vi "Main.vi"() -> ()   [LabVIEW 2014]
doc: "The boiler controller allows a user to start and shut down a boiler.\n\nUse the Reset, Start, and Light Pilot controls to sequentially start the boiler. \nUse the Fuel Control Valve to change the flow of fuel into the boiler. \nUse the Stop Boiler button to shut down the boiler. \nTo shut down the system or in the event of an emergency, use the Emergency Stop button to close the application completely."
uses:
  controls/MHL Data.ctl
  controls/MHL UI Data.ctl
  controls/MHL Status.ctl
  controls/MHL References.ctl
  controls/MHL Configuration.ctl
  support/Boiler System Globals.vi
  <vilib>/Utility/error.llb/Error Cluster From Error Code.vi
  <vilib>/ErrorRing/Error Ring.xnode
  support/Message Queue/Message Queue.lvlib
  support/User Event - Stop/User Event - Stop.lvlib
  Boiler/Boiler.lvlib
panel:
  in  "Fuel Control Valve":u32(slide) min=10 max=75 scale=10.0..75.0
  in  "Stop Boiler":bool
  in  "Light Pilot":bool
  out "Forced Draft Fan":bool
  out "Pilot":bool
  out "Pilot Gas Valve":bool
  out "Primary Fan":bool
  out "Status":string
  in  "Start":bool
  in  "Reset":bool
  in  "Emergency Stop":bool
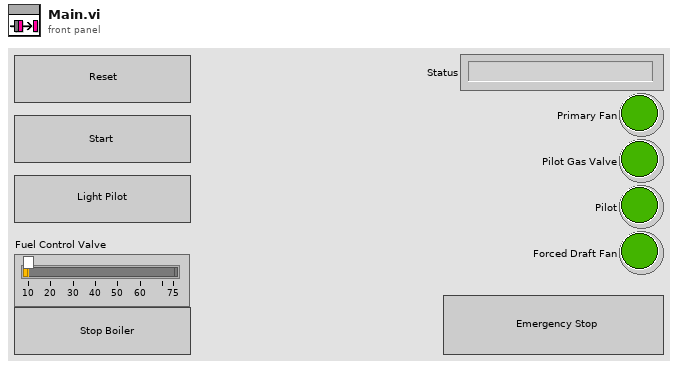
[diagram p1: front panel]
types:
  T1 = typedef "MHL Data.ctl" = cluster{"MHL User Interface Data":T2, "MHL References":T4, "MHL Configuration":T5}
  T2 = typedef "MHL UI Data.ctl" = cluster{"Status":string, "Fuel Control Valve":u32, "Primary Fan":bool, "Pilot Gas Valve":bool, "Pilot":bool, "Forced Draft Fan":bool, "MHL Status":T3}
  T3 = typedef "MHL Status.ctl" = enum16{"Lockout", "Ready", "Pre-Purge", "Pre-Purge Complete", "Pilot On", "Boiler Running", "Shutdown", "Purge"}
  T4 = typedef "MHL References.ctl" = cluster{"Reset Ref":refnum<vi>, "Start Ref":refnum<vi>, "Light Pilot Ref":refnum<vi>, "Stop Boiler Ref":refnum<vi>, "Fuel Control Valve Ref":refnum<vi>}
  T5 = typedef "MHL Configuration.ctl" = cluster{"Fuel Control Valve Maximum":dbl, "Fuel Control Valve Minimum":dbl}
  T6 = typedef "Notifiers.ctl" = cluster{"Handshake":refnum<notifier>, "Flame Level":refnum<notifier>, "Controller Exit":refnum<notifier>, "Boiler Exit":refnum<notifier>}
  T7 = typedef "Message Queue.lvlib/All Message Queues.ctl" = cluster{"MHL":refnum<queue>, "Boiler Controller":refnum<queue>, "Boiler":refnum<queue>}
  T8 = enum16{"open", "replace", "create", "open or create", "replace or create", "replace or create with confirmation"}
  T9 = enum32{"invalid app kind", "Development System", "Run Time System", "Student Edition", "Embedded LabVIEW", "Evaluation", "Custom"}
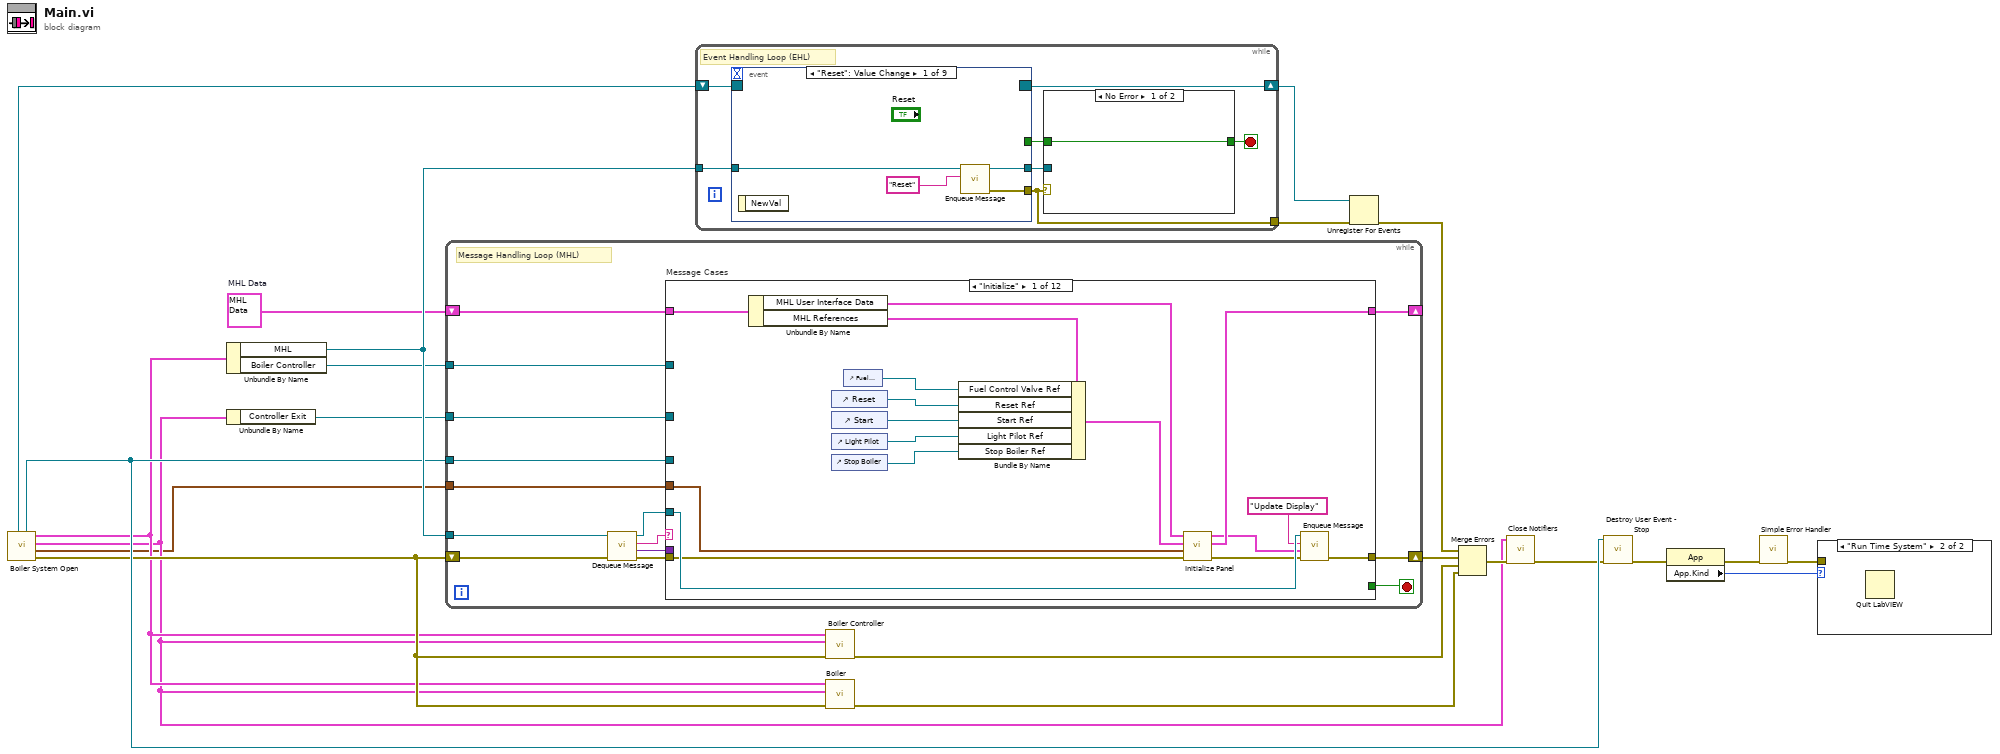
[diagram p0: block diagram]
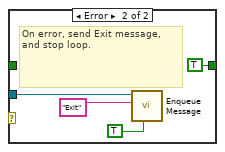
[diagram p3: hidden frame]
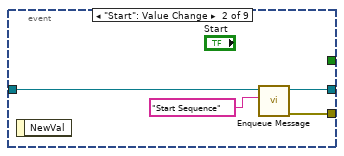
[diagram p4: hidden frame]
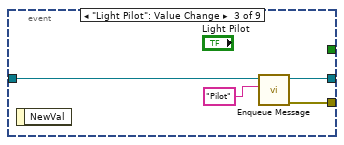
[diagram p5: hidden frame]
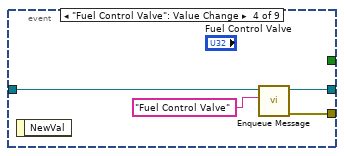
[diagram p6: hidden frame]
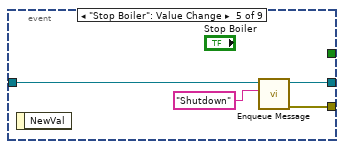
[diagram p7: hidden frame]
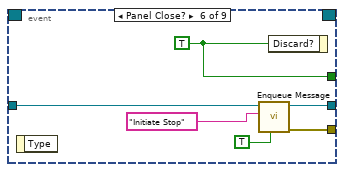
[diagram p8: hidden frame]
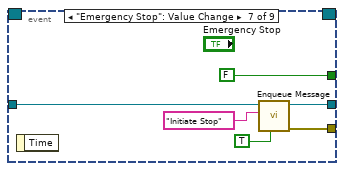
[diagram p9: hidden frame]
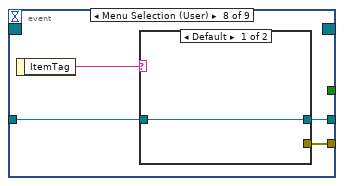
[diagram p10: hidden frame]
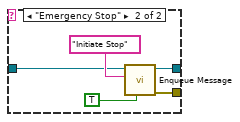
[diagram p11: hidden frame]
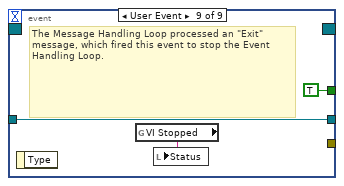
[diagram p12: hidden frame]
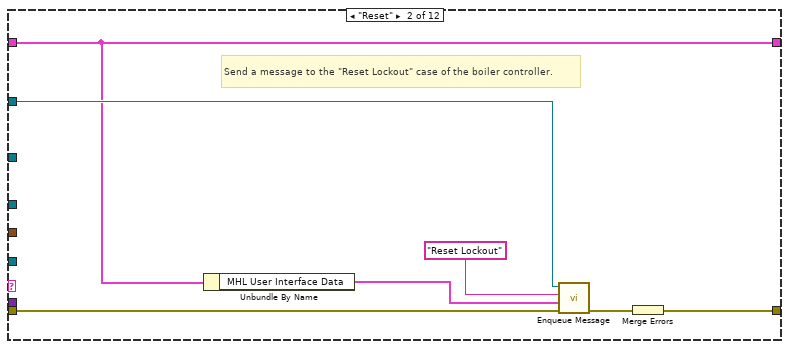
[diagram p13: hidden frame]
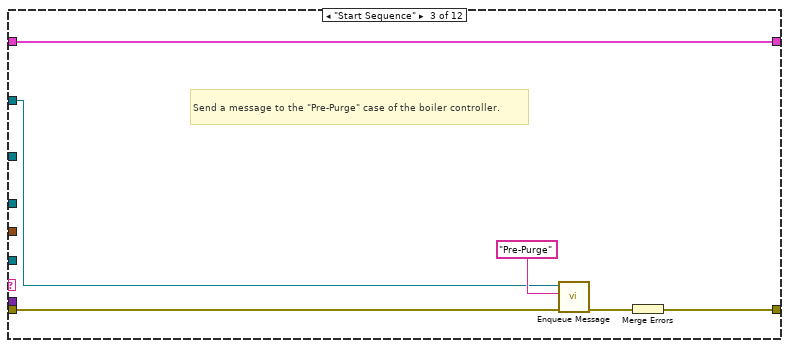
[diagram p14: hidden frame]
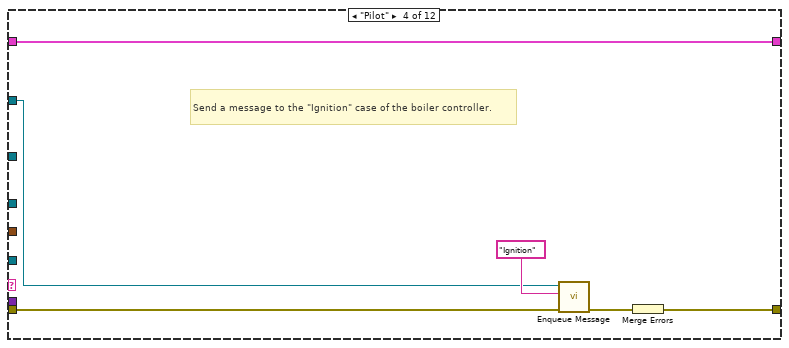
[diagram p15: hidden frame]
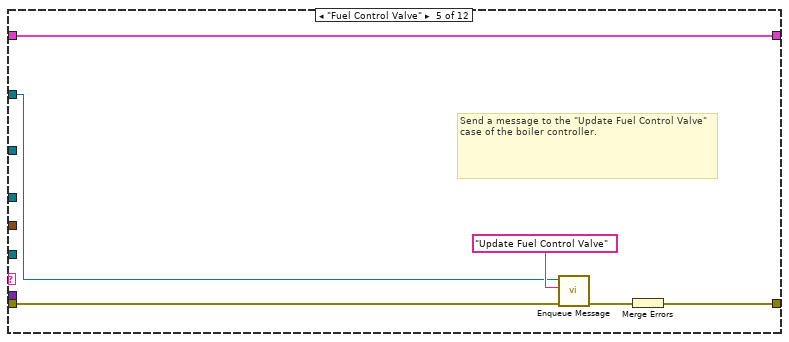
[diagram p16: hidden frame]
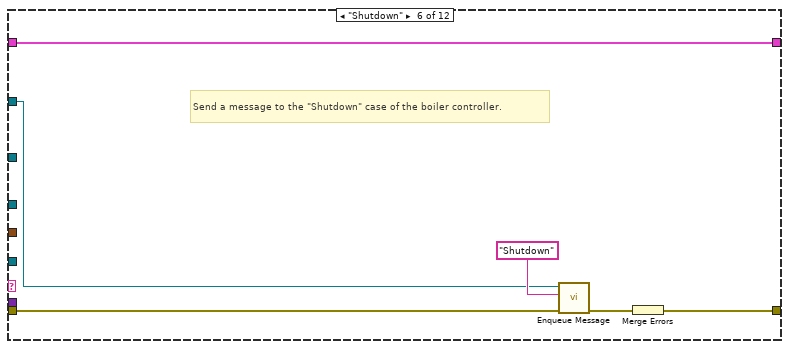
[diagram p17: hidden frame]
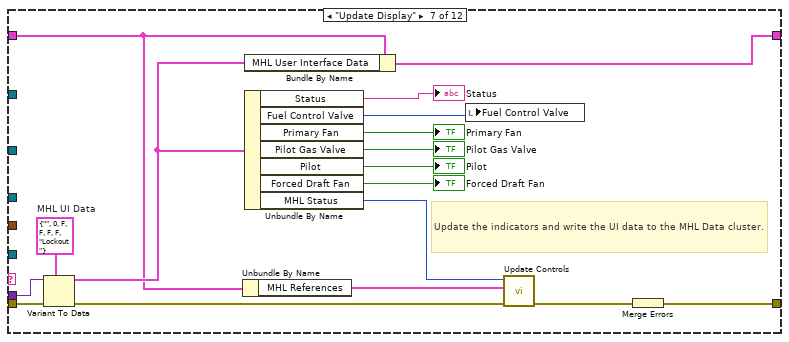
[diagram p18: hidden frame]
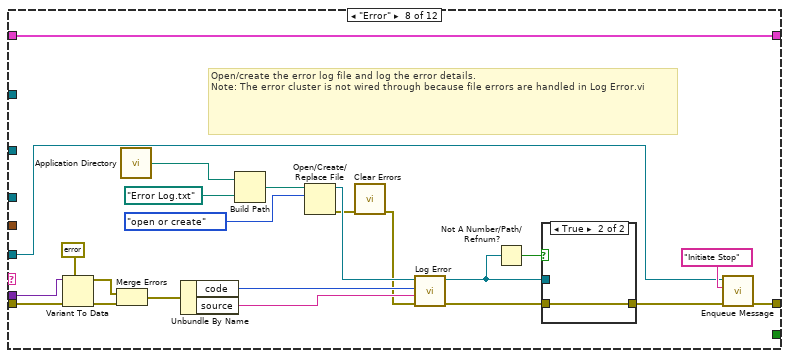
[diagram p19: hidden frame]
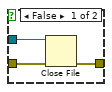
[diagram p20: hidden frame]
diagram:
  w16 = T1 {"MHL User Interface Data"={"Status"="", "Fuel Control Valve"=0, "Primary Fan"=FALSE, "Pilot Gas Valve"=FALSE, "Pilot"=FALSE, "Forced Draft Fan"=FALSE, "MHL Status"=enum."Lockout"}, "MHL References"={"Reset Ref"=refnum, "Start Ref"=refnum, "Light Pilot Ref"=refnum, "Stop Boiler Ref"=refnum, "Fuel Control Valve Ref"=refnum}, "MHL Configuration"={"Fuel Control Valve Maximum"=0.0, "Fuel Control Valve Minimum"=0.0}}  # MHL Data
  n1 = call "Boiler System Open.vi"() -> ("error out"=w7:errorcluster, "MHL Configuration"=w1:T5, "Notifiers"=w2:T6, "Message Queues"=w6:T7, "User Event - Stop"=w9:refnum<user-event>, "Stop Event Registration Refnum"=w10:refnum<event-registration>)  [unwired: 6 in]
  n2 = Unbundle By Name(w6) -> ("MHL"=w21:refnum<queue>, "Boiler Controller"=w14:refnum<queue>)
  n3 = Unbundle By Name(w2) -> ("Controller Exit"=w8:refnum<notifier>)
  n4 = while {
    tunnel: w21 -> [w26]
    shift-right: [w35] -> _
    shift-left: w16 -> [w36]
    tunnel: w9 -> [w32]
    shift-right: [w33] -> w22
    shift-left: w7 -> [w31]
    tunnel: w14 -> [w25]
    tunnel: w8 -> [w24]
    tunnel: w1 -> [w23]
    stop <- w34 stop-if-true
    # "Message Handling Loop (MHL)"
    n5 = call "Dequeue Message.vi"("error in (no error)"=w31, "Message Queue"=w26) -> ("error out"=w30:errorcluster, "Message Data"=w28:variant, "Message"=w29:string, "dup Message Queue"=w27:refnum<queue>)  [unwired: 6 in]
    n6 = case "Message Cases" shown="\"Initialize\"" w29 {
      selector: w29 -> [_ _ _ _ _ _ _ _ _ _ _ w162]
      tunnel: w27 -> [w46 _ _ _ _ _ _ w110 w131 w138 w160 _]
      tunnel: w30 -> [w40 w59 w64 w70 w73 w82 w100 w108 w136 w140 w153 _]
      tunnel: [w47 w60 w65 w71 w78 w83 w101 w106 w133 w139 w156 w161] -> w33
      tunnel: w36 -> [w48 w55 w66 w72 w74 w84 w86 w124 w135 w144 w159 w163]
      tunnel: [w38 w55 w66 w72 w74 w84 w90 w124 w135 w144 w159 w163] -> w35
      tunnel: [_ _ _ _ _ _ _ _ _ _ TRUE _] -> w34
      tunnel: w28 -> [_ _ _ _ _ _ w99 w107 _ _ _ _]
      tunnel: w32 -> [_ _ _ _ _ _ _ _ _ _ w155 _]
      tunnel: w25 -> [_ w56 w61 w67 w75 w79 _ _ w132 _ _ _]
      tunnel: w24 -> [_ _ _ _ _ _ _ _ _ w137 _ _]
      tunnel: w23 -> [w44 _ _ _ _ _ _ _ _ _ _ _]
      frame "Initialize" {
        n7 = Unbundle By Name(w48) -> ("MHL User Interface Data"=w41:T2, "MHL References"=w42:T4)
        n8 = control-ref of="Reset"() -> (w50:refnum<vi>)
        n9 = control-ref of="Start"() -> (w51:refnum<vi>)
        n10 = control-ref of="Light Pilot"() -> (w52:refnum<vi>)
        n11 = control-ref of="Stop Boiler"() -> (w53:refnum<vi>)
        n12 = control-ref of="Fuel Control Valve"() -> (w49:refnum<vi>)
        n13 = Bundle By Name(cluster=w42, "Fuel Control Valve Ref"=w49, "Reset Ref"=w50, "Start Ref"=w51, "Light Pilot Ref"=w52, "Stop Boiler Ref"=w53) -> (w43:T4)
        n14 = call "Initialize Panel.vi"("error in"=w40, "MHL Configuration"=w44, "MHL References"=w43, "MHL UI Data in"=w41) -> ("error out"=w39:errorcluster, "MHL Data out"=w38:T1, "MHL UI Data out"=w37:T2)  [unwired: 5 in]
        n15 = call "Enqueue Message.vi"("error in (no error)"=w39, "Message Data"=w37, "Message"="Update Display", "Message Queue"=w46) -> ("error out"=w47:errorcluster)  [unwired: 6 in, 1 out]
      }
      frame "Reset" {
        # "Send a message to the \"Reset Lockout\" case of the boiler controller."
        n16 = Unbundle By Name(w55) -> ("MHL User Interface Data"=w54:T2)
        n17 = call "Enqueue Message.vi"("error in (no error)"=w59, "Message Data"=w54, "Message"="Reset Lockout", "Message Queue"=w56) -> ("error out"=w58:errorcluster)  [unwired: 6 in, 1 out]
        n18 = Merge Errors(w58) -> (w60:errorcluster)
      }
      frame "Start Sequence" {
        # "Send a message to the \"Pre-Purge\" case of the boiler controller."
        n19 = call "Enqueue Message.vi"("error in (no error)"=w64, "Message"="Pre-Purge", "Message Queue"=w61) -> ("error out"=w63:errorcluster)  [unwired: 7 in, 1 out]
        n20 = Merge Errors(w63) -> (w65:errorcluster)
      }
      frame "Pilot" {
        # "Send a message to the \"Ignition\" case of the boiler controller."
        n21 = call "Enqueue Message.vi"("error in (no error)"=w70, "Message"="Ignition", "Message Queue"=w67) -> ("error out"=w69:errorcluster)  [unwired: 7 in, 1 out]
        n22 = Merge Errors(w69) -> (w71:errorcluster)
      }
      frame "Fuel Control Valve" {
        # "Send a message to the \"Update Fuel Control Valve\" case of the boiler controller."
        n23 = call "Enqueue Message.vi"("error in (no error)"=w73, "Message"="Update Fuel Control Valve", "Message Queue"=w75) -> ("error out"=w77:errorcluster)  [unwired: 7 in, 1 out]
        n24 = Merge Errors(w77) -> (w78:errorcluster)
      }
      frame "Shutdown" {
        # "Send a message to the \"Shutdown\" case of the boiler controller."
        n25 = call "Enqueue Message.vi"("error in (no error)"=w82, "Message"="Shutdown", "Message Queue"=w79) -> ("error out"=w81:errorcluster)  [unwired: 7 in, 1 out]
        n26 = Merge Errors(w81) -> (w83:errorcluster)
      }
      frame "Update Display" {
        w98 = T2 {"Status"="", "Fuel Control Valve"=0, "Primary Fan"=FALSE, "Pilot Gas Valve"=FALSE, "Pilot"=FALSE, "Forced Draft Fan"=FALSE, "MHL Status"=enum."Lockout"}  # MHL UI Data
        # "Update the indicators and write the UI data to the MHL Data cluster."
        n27 = Variant To Data(error in=w100, type=w98, Variant=w99) -> (data=w91:T2, error out=w89:errorcluster)
        n28 = Unbundle By Name(w86) -> ("MHL References"=w85:T4)
        n29 = Bundle By Name(cluster=w86, "MHL User Interface Data"=w91) -> (w90:T1)
        n30 = Unbundle By Name(w91) -> ("Status"=→"Status":string, "Fuel Control Valve"=w96:u32, "Primary Fan"=→"Primary Fan":bool, "Pilot Gas Valve"=→"Pilot Gas Valve":bool, "Pilot"=→"Pilot":bool, "Forced Draft Fan"=→"Forced Draft Fan":bool, "MHL Status"=w87:T3)
        n31 = local write "Fuel Control Valve"(w96) -> ()
        n32 = call "Update Controls.vi"("error in"=w89, "MHL References"=w85, "MHL Status"=w87) -> ("error out"=w88:errorcluster)  [unwired: 8 in]
        n33 = Merge Errors(w88) -> (w101:errorcluster)
      }
      frame "Error" {
        # "Open/create the error log file and log the error details.\nNote: The error cluster is not wired through because file errors are handled in Log Error.vi"
        n34 = Variant To Data(error in=w108, type=errorcluster {"status"=FALSE, "code"=0, "source"=""} ("error out"), Variant=w107) -> (data=w120:errorcluster, error out=w121:errorcluster)
        n35 = Merge Errors(w120, w121) -> (w119:errorcluster)
        n36 = call <vilib>:"Application Directory.vi"() -> ("Application Directory"=w118:path)
        n37 = Unbundle By Name(w119) -> ("code"=w113:i32, "source"=w112:string)
        n38 = Build Path(base path=w118, name or relative path=path "Error Log.txt") -> (appended path=w117:path)
        n39 = Open/Create/Replace File(file path (use dialog)=w117, operation (0:open)=T8."open or create") -> (refnum out=w115:refnum<file>, error out=w103:errorcluster)  [unwired: 4 in, 1 out]
        n40 = call <vilib>:"Clear Errors.vi"("error in (no error)"=w103) -> ("error out"=w102:errorcluster)  [unwired: 5 in, 1 out]
        n41 = call "Log Error.vi"("error in"=w102, "Source"=w112, "Code"=w113, "Error Log Refnum In"=w115) -> ("error out"=w114:errorcluster, "Error Log Refnum Out"=w105:refnum<file>)  [unwired: 6 in]
        n42 = Not A Number/Path/Refnum?(number/path/refnum=w105) -> (NaN/Path/Refnum?=w104:bool)
        n43 = case shown="True" w104 {
          tunnel: w114 -> [w127 w128]
          tunnel: w105 -> [w126 _]
          tunnel: [w125 w128] -> w111
          frame False {
            n44 = Close File(refnum=w126, error in=w127) -> (error out=w125:errorcluster)  [unwired: 1 out]
          }
          frame True {
          }
        }
        n45 = call "Enqueue Message.vi"("error in (no error)"=w111, "Message"="Initiate Stop", "Message Queue"=w110) -> ("error out"=w106:errorcluster)  [unwired: 7 in, 1 out]
      }
      frame "Initiate Stop" {
        # "When stopping, first send a message to stop the boiler controller. Then wait for the boiler and boiler controller to exit."
        n46 = call "Enqueue Message.vi"("error in (no error)"=w136, "Message"="Exit", "Message Queue"=w132) -> ("error out"=w134:errorcluster)  [unwired: 7 in, 1 out]
        n47 = call "Enqueue Message.vi"("error in (no error)"=w134, "Message"="Wait on Boiler Exit", "Message Queue"=w131) -> ("error out"=w133:errorcluster)  [unwired: 7 in, 1 out]
      }
      frame "Wait on Boiler Exit" {
        # "Monitor the boiler controller to determine if it has completed its Exit. Wait 10 milliseconds for the boiler controller to respond. \nIf the notification does not occur, then enqueue another Wait on Boiler Exit message.\nIf the notification occurs, then exit the Message Handling Loop."
        n48 = Wait on Notification(notifier=w137, timeout in ms (-1)=10, error in (no error)=w140) -> (timed out?=w142:bool, error out=w141:errorcluster)  [unwired: 1 in, 2 out]
        n49 = case shown="True" w142 {
          tunnel: w141 -> [w148 w152]
          tunnel: w138 -> [w147 w150]
          tunnel: [w145 w151] -> w139
          frame False {
            n50 = call "Enqueue Message.vi"("error in (no error)"=w148, "Message"="Exit", "Message Queue"=w147) -> ("error out"=w145:errorcluster)  [unwired: 7 in, 1 out]
          }
          frame True {
            n51 = call "Enqueue Message.vi"("error in (no error)"=w152, "Message"="Wait on Boiler Exit", "Message Queue"=w150) -> ("error out"=w151:errorcluster)  [unwired: 7 in, 1 out]
          }
        }
      }
      frame "Exit" {
        # "Stop the VI"
        # "Release the message queue reference"
        n52 = call "Fire User Event - Stop.vi"("User Event - Stop"=w155) -> ("error out"=w154:errorcluster)  [unwired: 10 in]
        n53 = Release Queue(queue=w160, error in (no error)=w153) -> (error out=w157:errorcluster)  [unwired: 1 in, 2 out]
        n54 = Merge Errors(w154, w157) -> (w156:errorcluster)
      }
      frame Default {
        # "'Default' case only runs if there is a message that isn't defined in any of the other cases.  Output a programming error."
        n55 = xnode "Error Ring"("parameter 0"=w162) -> ("error out"=w161:errorcluster)
      }
    }
  }
  n56 = while {
    tunnel: w21 -> [w177]
    tunnel: [w173] -> w18
    shift-right: [w171] -> w17
    shift-left: w10 -> [w172]
    stop <- w175 stop-if-true
    # "Event Handling Loop (EHL)"
    n57 = event shown="[0] \"Reset\": Value Change" {
      selector: w172 -> [_ _ _ _ _ _ _ _ _]
      dyn-events: [_ _ _ _ _ _ _ _ _] -> w171
      timeout: _ -> [_ _ _ _ _ _ _ _ _]
      tunnel: [_ _ _ _ _ w208 FALSE ("Discard?") _ TRUE ("Discard?")] -> w176
      tunnel: w177 -> [w186 w190 w194 w198 w202 w207 w214 w217 w227]
      tunnel: [w185 w188 w192 w196 w200 w206 w213 w215 _] -> w173
      tunnel: [w184 w189 w193 w197 w201 w205 w211 w216 w227] -> w174
      event "Reset": Value Change {
        n58 = event-data() -> ()  [unwired: 1 in, 1 out]
        n59 = call "Enqueue Message.vi"("Message"="Reset", "Message Queue"=w186) -> ("error out"=w185:errorcluster, "dup Message Queue"=w184:refnum<queue>)  [unwired: 8 in]
      }
      event "Start": Value Change {
        n60 = event-data() -> ()  [unwired: 1 in, 1 out]
        n61 = call "Enqueue Message.vi"("Message"="Start Sequence", "Message Queue"=w190) -> ("error out"=w188:errorcluster, "dup Message Queue"=w189:refnum<queue>)  [unwired: 8 in]
      }
      event "Light Pilot": Value Change {
        n62 = event-data() -> ()  [unwired: 1 in, 1 out]
        n63 = call "Enqueue Message.vi"("Message"="Pilot", "Message Queue"=w194) -> ("error out"=w192:errorcluster, "dup Message Queue"=w193:refnum<queue>)  [unwired: 8 in]
      }
      event "Fuel Control Valve": Value Change {
        n64 = event-data() -> ()  [unwired: 1 in, 1 out]
        n65 = call "Enqueue Message.vi"("Message"="Fuel Control Valve", "Message Queue"=w198) -> ("error out"=w196:errorcluster, "dup Message Queue"=w197:refnum<queue>)  [unwired: 8 in]
      }
      event "Stop Boiler": Value Change {
        n66 = event-data() -> ()  [unwired: 1 in, 1 out]
        n67 = call "Enqueue Message.vi"("Message"="Shutdown", "Message Queue"=w202) -> ("error out"=w200:errorcluster, "dup Message Queue"=w201:refnum<queue>)  [unwired: 8 in]
      }
      event Panel Close? {
        w208 = TRUE ("Discard?")
        n68 = event-data() -> ()  [unwired: 1 in, 1 out]
        n69 = call "Enqueue Message.vi"("Priority Message? (F)"=TRUE, "Message"="Initiate Stop", "Message Queue"=w207) -> ("error out"=w206:errorcluster, "dup Message Queue"=w205:refnum<queue>)  [unwired: 7 in]
        n70 = event-data("Discard?"=w208) -> ()  [unwired: 1 in, 1 out]
      }
      event "Emergency Stop": Value Change {
        n71 = event-data() -> ()  [unwired: 1 in, 1 out]
        n72 = call "Enqueue Message.vi"("Priority Message? (F)"=TRUE, "Message"="Initiate Stop", "Message Queue"=w214) -> ("error out"=w213:errorcluster, "dup Message Queue"=w211:refnum<queue>)  [unwired: 7 in]
      }
      event Menu Selection (User) {
        n73 = event-data() -> ("ItemTag"=w218:string)  [unwired: 1 in]
        n74 = case shown="Default" w218 {
          tunnel: w217 -> [w219 w222]
          tunnel: [w219 w221] -> w216
          tunnel: [_ w220] -> w215
          frame Default {
          }
          frame "Emergency Stop" {
            n75 = call "Enqueue Message.vi"("Priority Message? (F)"=TRUE, "Message"="Initiate Stop", "Message Queue"=w222) -> ("error out"=w220:errorcluster, "dup Message Queue"=w221:refnum<queue>)  [unwired: 7 in]
          }
        }
      }
      event User Event {
        # "The Message Handling Loop processed an \"Exit\" message, which fired this event to stop the Event Handling Loop."
        n76 = event-data() -> ()  [unwired: 1 in, 1 out]
        n77 = global read "Boiler System Globals.vi" "VI Stopped"() -> (w225:string)
        n78 = local write "Status"(w225) -> ()
      }
    }
    n79 = case shown="No Error" w173 {
      tunnel: [w178 TRUE ("Discard?")] -> w175
      tunnel: w176 -> [w178 _]
      tunnel: w174 -> [_ w181]
      frame No Error {
      }
      frame Error {
        # "On error, send Exit message, and stop loop."
        n80 = call "Enqueue Message.vi"("Priority Message? (F)"=TRUE, "Message"="Exit", "Message Queue"=w181) -> ()  [unwired: 7 in, 2 out]
      }
    }
  }
  n81 = call "Boiler Controller.vi"("error in"=w7, "Notifiers"=w2, "Message Queues"=w6) -> ("error out"=w15:errorcluster)  [unwired: 8 in]
  n82 = call "Boiler.vi"("error in"=w7, "Notifiers"=w2, "Message Queues"=w6) -> ("error out"=w5:errorcluster)  [unwired: 8 in]
  n83 = Unregister For Events(event registration refnum=w17, error in=w18) -> (error out=w19:errorcluster)
  n84 = Merge Errors(w19, w22, w15, w5) -> (w4:errorcluster)
  n85 = call "Close Notifiers.vi"("error in"=w4, "Notifiers"=w2) -> ("error out"=w3:errorcluster)  [unwired: 9 in]
  n86 = call "Destroy User Event - Stop.vi"("error in (no error)"=w3, "User Event - Stop"=w9) -> ("error out"=w20:errorcluster)  [unwired: 9 in]
  n87 = property class="App"(error in=w20) -> (error out=w13:errorcluster, "App.Kind"=w12:T9)  [unwired: 1 in, 1 out]
  n88 = call <vilib>:"Simple Error Handler.vi"("error in (no error)"=w13) -> ("error out"=w11:errorcluster)  [unwired: 4 in, 4 out]
  n89 = case shown="\"Run Time System\"" w12 {
    tunnel: w11 -> [_ _]
    frame Default {
    }
    frame "Run Time System" {
      n90 = Quit LabVIEW() -> ()  [unwired: 1 in]
    }
  }
